vi "HandleClapper.vi"(7 "InitState":T1=enum."Middle", 8 "error in (no error)":errorcluster, 11 "Toggle?":bool) -> (0 "error out":errorcluster, 2 "State":T1, 3 "Enqueue?":bool)   [LabVIEW 2013]
uses:
  DoubleSolenoidAction.ctl
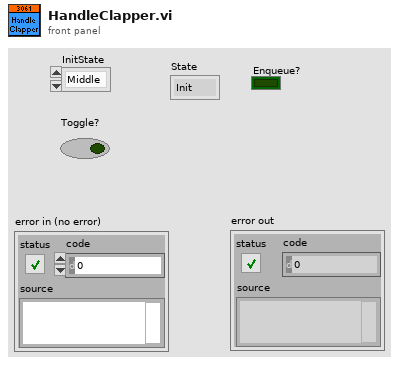
[diagram p1: front panel]
types:
  T1 = typedef "DoubleSolenoidAction.ctl" = enum16{"Init", "Middle", "In", "Out"}
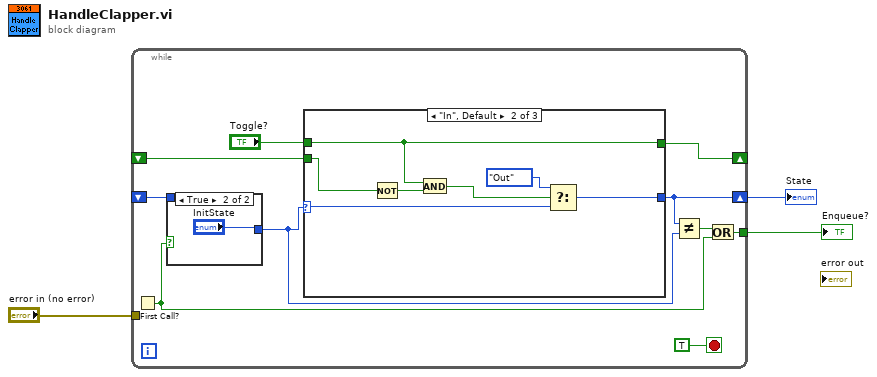
[diagram p0: block diagram]
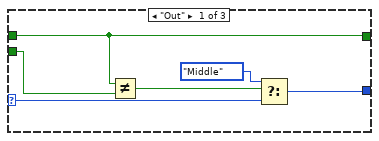
[diagram p3: hidden frame]
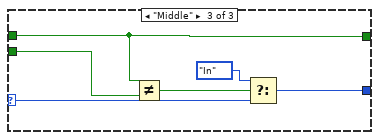
[diagram p4: hidden frame]
diagram:
  n1 = while {
    shift-right: [w5] -> w2
    shift-left: _ -> [w9]
    shift-right: [w11] -> _
    shift-left: _ -> [w10]
    tunnel: "error in (no error)" -> [_]
    tunnel: [w6] -> w1
    stop <- TRUE stop-if-true
    n2 = First Call?() -> (First Call?: T/F=w8:bool)
    n3 = case shown="True" w8 {
      tunnel: [w14 "InitState"] -> w4
      tunnel: w9 -> [w14 _]
      frame False {
      }
      frame True {
      }
    }
    n4 = case shown="\"In\", Default" w4 {
      selector: w4 -> [w19 w26 w34]
      tunnel: [w20 w27 w33] -> w5
      tunnel: [w16 w25 w31] -> w11
      tunnel: "Toggle?" -> [w16 w25 w31]
      tunnel: w10 -> [w17 w22 w30]
      frame "Out" {
        n5 = Not Equal?(x=w16, y=w17) -> (x != y?=w18:bool)
        n6 = Select(t=DoubleSolenoidAction."Middle", s=w18, f=w19) -> (s? t:f=w20:T1)
      }
      frame "In", Default {
        n7 = Not(x=w22) -> (.not. x?=w23:bool)
        n8 = And(x=w25, y=w23) -> (x .and. y?=w24:bool)
        n9 = Select(t=DoubleSolenoidAction."Out", s=w24, f=w26) -> (s? t:f=w27:T1)
      }
      frame "Middle" {
        n10 = Not Equal?(x=w31, y=w30) -> (x != y?=w29:bool)
        n11 = Select(t=DoubleSolenoidAction."In", s=w29, f=w34) -> (s? t:f=w33:T1)
      }
    }
    n12 = Not Equal?(x=w5, y=w4) -> (x != y?=w7:bool)
    n13 = Or(x=w7, y=w8) -> (x .or. y?=w6:bool)
  }
  "State" <- w2
  "Enqueue?" <- w1
